vi "TestOK.vi"() -> ()   [LabVIEW 2020]
panel:
  out "arrayout":dbl[](array[numeric])=[1.0, 2.0]
  in  "arrayin":dbl[](array[numeric])=[1.0, 2.0]
  out "booleanoutprivate":bool
  in  "booleaninprivate":bool
  out "time":dbl
  in  "doublein":dbl(slide)=1.0101010101010104 scale=-100.0..100.0
  out "doubleout":dbl=1.0101
  in  "stringin":string="hello"
  in  "booleanin":bool
  out "booleanout":bool
  out "stringout":string="hello"
  in  "stop":bool
  out "intout":i32=5
  in  "intin":i32=5
  # "Note there is one control and  one indicator \nthat are hidden (booleaninprivate and \nbooleanoutprivate)!"
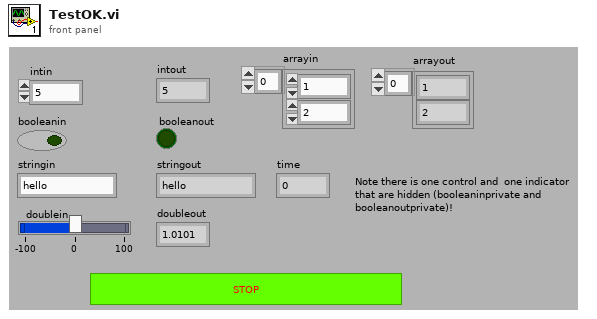
[diagram p1: front panel]
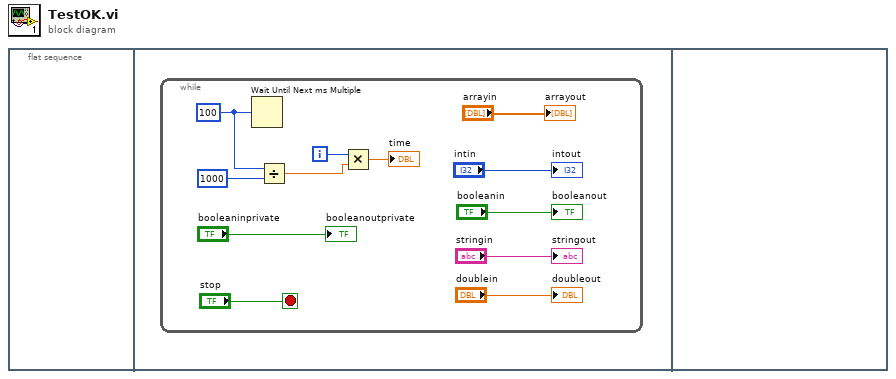
[diagram p0: block diagram]
diagram:
  n1 = flat-sequence {
    frame #0 {
    }
    frame #1 {
      n2 = while {
        i -> [w7]
        stop <- "stop" stop-if-true
        w8 = u32 100 ("millisecond multiple")
        n3 = Wait Until Next ms Multiple(millisecond multiple=w8) -> ()  [unwired: 1 out]
        n4 = Divide(x=w8, y=i64 1000) -> (x/y=w10:dbl)
        n5 = Multiply(x=w7, y=w10) -> (x*y=→"time":dbl)
        "intout" <- "intin"
        "stringout" <- "stringin"
        "booleanout" <- "booleanin"
        "doubleout" <- "doublein"
        "booleanoutprivate" <- "booleaninprivate"
        "arrayout" <- "arrayin"
      }
    }
    frame #2 {
    }
  }
